vi "Servo_control.vi"(11 "Slide in":dbl(slide) scale=0.0..168.0) -> (0 "error out":errorcluster, 2 "Angle":dbl, 3 "Duty cycle":dbl)   [LabVIEW 2021]
uses:
  PWM_channel_list.ctl
  <vilib>/Utility/error.llb/Error Cluster From Error Code.vi
  <vilib>/myRIO/Common/Instrument Driver Framework/myRIO v1.0/PWM/vis/myRIO v1.0 Write PWM.vi
  <vilib>/myRIO/Instrument Drivers/Onboard IO/PWM/PWM.lvlib
panel:
  in  "Channel Name":T1
  in  "error in (no error)":errorcluster
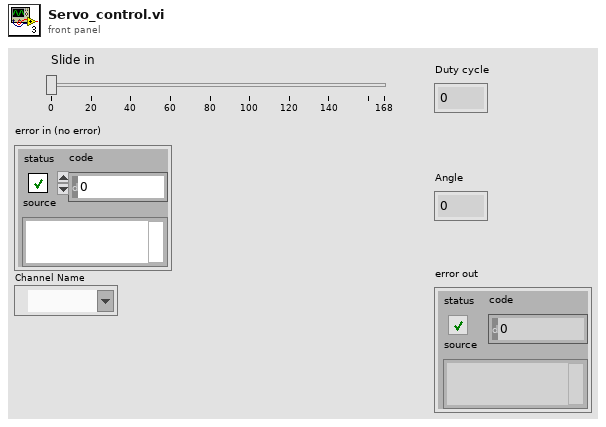
[diagram p1: front panel]
types:
  T1 = typedef "PWM_channel_list.ctl" = tag
  T2 = typedef "PWM.lvlib/PWM Reference.ctl" = cluster{"myRIO Reference":T3, "PWM Channels Enum":T7, "PWM Configuration":T8}
  T3 = typedef "myRIO Generic Hardware Reference.ctl" = cluster{"myRIO Model":T4, "myRIO Hardware Reference":T5}
  T4 = typedef "Hardware Version Enum.ctl" = enum16{"Unknown", "myRIO-1900", "myRIO-1950", "roboRIO", "NI ELVIS RIO CM", "ELVIS III"}
  T5 = typedef "myRIO v1.0 Reference.ctl" = cluster{"Generic FPGA Reference":T6, "Allow multiple opens":bool}
  T6 = typedef "Generic FPGA Reference.ctl" = refnum<k20>
  T7 = typedef "PWM Channels Enum.ctl" = enum16{"Not Connected", "C/PWM0", "C/PWM1", "A/PWM0", "A/PWM1", "A/PWM2", "A/PWM3", "A/PWM4", "A/PWM5", "A/PWM6", "A/PWM7", "A/PWM8", "A/PWM9", "A/PWM10", "A/PWM11", "A/PWM12", "A/PWM13", "A/PWM14", "A/PWM15", "A/PWM16", "A/PWM17", "A/PWM18", "A/PWM19", "B/PWM0", "B/PWM1", "B/PWM2", "B/PWM3", "B/PWM4", "B/PWM5", "B/PWM6", "B/PWM7", "B/PWM8", "B/PWM9", "B/PWM10", "B/PWM11", "B/PWM12", "B/PWM13", "B/PWM14", "B/PWM15", "B/PWM16", "B/PWM17", "B/PWM18", "B/PWM19", "PWM/PWM0", "PWM/PWM1", "PWM/PWM2", "PWM/PWM3", "PWM/PWM4", "PWM/PWM5", "PWM/PWM6", "PWM/PWM7", "PWM/PWM8", "PWM/PWM9"}
  T8 = typedef "PWM.lvlib/PWM Configuration.ctl" = cluster{"Frequency":dbl, "Duty Cycle":dbl}
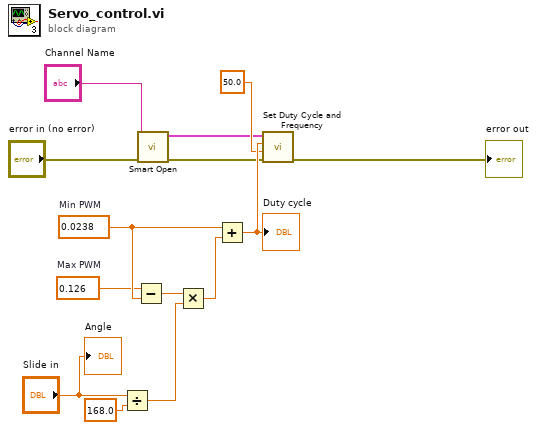
[diagram p0: block diagram]
diagram:
  w3 = 0.126  # Max PWM
  w6 = 0.0238  # Min PWM
  n1 = Divide(x="Slide in", y=168.0 ("x")) -> (x/y=w8:dbl)
  n2 = Subtract(x=w3, y=w6) -> (x-y=w4:dbl)
  n3 = call <vilib>:"Smart Open.vi"("error in (no error)"="error in (no error)", "Channel Name"="Channel Name") -> ("error out"=w13:errorcluster, "PWM Ref Out"=w10:T2)  [unwired: 8 in]
  n4 = Multiply(x=w4, y=w8) -> (x*y=w5:dbl)
  n5 = Add(x=w6, y=w5) -> (x+y=w14:dbl)
  "Duty cycle" <- w14
  n6 = call <vilib>:"Set Duty Cycle and Frequency.vi"("error in (no error)"=w13, "Frequency [Hz]"=50.0, "Duty Cycle"=w14, "PWM Ref In"=w10) -> ("error out"=→"error out":errorcluster)  [unwired: 5 in, 1 out]
  "Angle" <- "Slide in"
